vi "FLT_addation.vi"(1 "y":dbl, 2 "x":dbl) -> (0 "x+y":dbl)   [LabVIEW 2020]
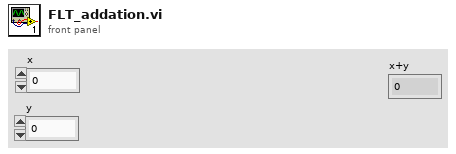
[diagram p1: front panel]
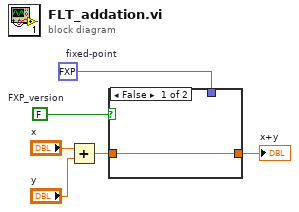
[diagram p0: block diagram]
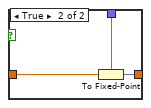
[diagram p2: hidden frame]
diagram:
  w1 = fxp<+,1,1> 0.0  # fixed-point
  w2 = FALSE  # FXP_version
  n1 = Add(x="x", y="y") -> (x+y=w3:dbl)
  n2 = case shown="False" w2 {
    tunnel: [w7 w10] -> w4
    tunnel: w3 -> [w7 w9]
    tunnel: w1 -> [_ w8]
    frame False {
    }
    frame True {
      n3 = To Fixed-Point(fixed-point type=w8, number=w9) -> (fixed-point=w10:fxp<+,1,1>)
    }
  }
  "x+y" <- w4
